vi "executePlayVSS.vi"(8 "error in (no error)":errorcluster, 11 "Game in":refnum<class "Game.lvclass">) -> (0 "error out":errorcluster, 3 "Game out":refnum<class "Game.lvclass">)   [LabVIEW 2020, in "Game.lvclass"]
uses:
  Game.lvclass
  Utilities_class/Utilities.lvclass
  HaltRole_class/HaltRole.lvclass
  AttackerAimGoalRoleVSS_class/AttackerAimGoalRoleVSS.lvclass
  Playbook_class/Playbook.lvclass
  BallChallengerAttackerRoleVSS_class/BallChallengerAttackerRoleVSS.lvclass
  KeeperRoleVSS_class/KeeperRoleVSS.lvclass
  NormalAttackerRoleVSS_class/NormalAttackerRoleVSS.lvclass
  DefenderAreaRoleVSS_class/DefenderAreaRoleVSS.lvclass
  TimeoutRole_class/TimeoutRole.lvclass
  PrepareFreeBallPlayVSS_class/PrepareFreeBallPlayVSS.lvclass
  PrepareGoalKickEnemyPlayVSS_class/PrepareGoalKickEnemyPlayVSS.lvclass
  Ally_class/Ally.lvclass
  TimeoutPlay_class/TimeoutPlay.lvclass
  DeadBallPlayVSS_class/DeadBallPlayVSS.lvclass
  NormalGamePlayVSS_class/NormalGamePlayVSS.lvclass
  PreparePenaltyAllyPlayVSS_class/PreparePenaltyAllyPlayVSS.lvclass
  HaltPlay_class/HaltPlay.lvclass
  BallChallengePlayVSS_class/BallChallengePlayVSS.lvclass
  PenaltyEnemyPlayVSS_class/PenaltyEnemyPlayVSS.lvclass
  KickPenaltyAllyPlayVSS_class/KickPenaltyAllyPlayVSS.lvclass
  Robot_class/Robot.lvclass
  PrepareGoalKickAllyPlayVSS_class/PrepareGoalKickAllyPlayVSS.lvclass
  PrepareKickoffAllyPlayVSS_class/PrepareKickoffAllyPlayVSS.lvclass
  PreparePenaltyEnemyPlayVSS_class/PreparePenaltyEnemyPlayVSS.lvclass
  PrepareKickoffEnemyPlay_class/PrepareKickoffEnemyPlay.lvclass
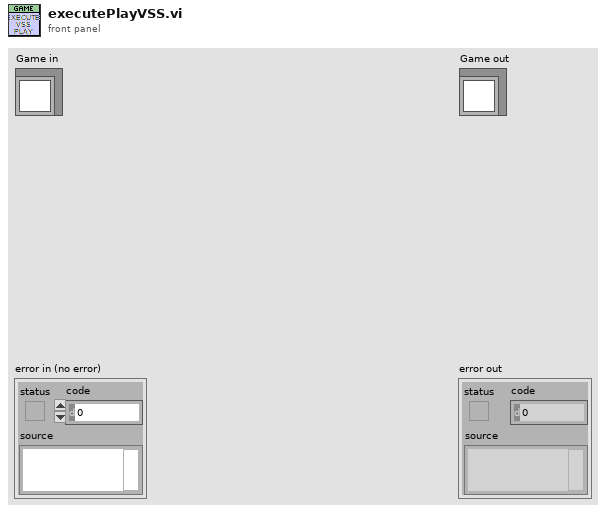
[diagram p1: front panel]
types:
  T1 = cluster{"id":i32, "x":dbl, "y":dbl, "orientation":dbl}[]
  T2 = enum16{"FreeBall", "PrepareFreeBall", "GoalKickEnemy", "GoalKickAlly", "KickoffAlly", "KickoffEnemy", "PrepareGoalKickEnemy", "PrepareGoalKickAlly", "Stop", "PrepareKickoffEnemy", "PrepareKickoffAlly", "PreparePenaltyEnemy", "Timeout", "DeadBall", "NormalGame", "KickPenaltyAlly", "PenaltyEnemy", "BallChallenge", "PreparePenaltyAlly", "Halt"}
  T3 = typedef "offensive_plays.ctl" = cluster{"Play":refnum<class "Play.lvclass">, "TestPlay":refnum<class "TestPlay.lvclass">, "EnemyPossessionAtEnemyFieldPlay":refnum<class "EnemyPossessionAtEnemyFieldPlay.lvclass">, "EnemyPossessionAtOurFieldPlay":refnum<class "EnemyPossessionAtOurFieldPlay.lvclass">, "NormalGamePlay":refnum<class "NormalGamePlay.lvclass">, "IndirectEnemyPlay":refnum<class "IndirectEnemyPlay.lvclass">, "PrepareKickoffAllyPlay":refnum<class "PrepareKickoffAllyPlay.lvclass">, "PrepareKickoffEnemyPlay":refnum<class "PrepareKickoffEnemyPlay.lvclass">, "KickPenaltyAllyPlay":refnum<class "KickPenaltyAllyPlay.lvclass">, "PreparePenaltyAllyPlay":refnum<class "PreparePenaltyAllyPlay.lvclass">, "DirectEnemyPlay":refnum<class "DirectEnemyPlay.lvclass">, "PreparePenaltyEnemyPlay":refnum<class "PreparePenaltyEnemyPlay.lvclass">, "BallOutOfFieldPlay":refnum<class "BallOutOfFieldPlay.lvclass">, "StopOffensivePlay":refnum<class "StopOffensivePlay.lvclass">, "PassPlay":refnum<class "PassPlay.lvclass">, "DirectKickPlay":refnum<class "DirectKickPlay.lvclass">, "HaltPlay":refnum<class "HaltPlay.lvclass">, "PreparePassPlay":refnum<class "PreparePassPlay.lvclass">, "PassToStrikerPlay":refnum<class "PassToStriker.lvclass">, "PassTo2ndStrikerPlay":refnum<class "PassTo2ndStriker.lvclass">, "SimplePassPlay":refnum<class "SimplePass.lvclass">, "PrepareRollToPassPlay":refnum<class "PrepareRollToPassPlay.lvclass">, "PrepareDoublePassPlay":refnum<class "PrepareDoublePassPlay.lvclass">, "TableWith2ndStrikerPlay":refnum<class "TableWith2ndStrikerPlay.lvclass">, "TableWithStrikerPlay":refnum<class "TableWithStrikerPlay.lvclass">}
  T4 = typedef "roles.ctl" = enum16{"BallChallengerAttackerVSS", "NormalAttackerVSS", "AttackerAimGoalVSS", "DefenderAreaVSS", "KeeperVSS", "Tabler", "TableFinalizer", "PrepareRollToPassRoller", "PrepareRollToPassReceiver", "SimplePassRoll", "SimplePassRollReceiver", "PenaltyDefense", "PreparePassReceiver 2", "PreparePassReceiver 1", "PassObserver", "Timeout", "Goto", "ZigZag", "None", "BallOutOfField", "DefenderArea", "Duelist", "AttackerStop", "FollowAttacker", "KeeperRole", "KickPenalty", "AttackerAimGoal", "AttackerBlock", "Marker", "Halt", "Shoot", "PassKicker", "PassReceiver", "TestRole", "PenaltyAttacker"}
  T5 = cluster{"HaltRole 1":refnum<class "HaltRole.lvclass">, "HaltRole 2":refnum<class "HaltRole.lvclass">, "HaltRole 3":refnum<class "HaltRole.lvclass">, "HaltRole 4":refnum<class "HaltRole.lvclass">, "HaltRole 5":refnum<class "HaltRole.lvclass">, "HaltRole 6":refnum<class "HaltRole.lvclass">}
  T6 = cluster{"PreparePenaltyAllyPlayVSS":refnum<class "PreparePenaltyAllyPlayVSS.lvclass">, "HaltPlay":refnum<class "HaltPlay.lvclass">, "DeadBallPlayVSS":refnum<class "DeadBallPlayVSS.lvclass">, "NormalGamePlayVSS":refnum<class "NormalGamePlayVSS.lvclass">, "BallChallengePlayVSS":refnum<class "BallChallengePlayVSS.lvclass">, "PenaltyEnemyPlayVSS":refnum<class "PenaltyEnemyPlayVSS.lvclass">, "TimeoutPlay":refnum<class "TimeoutPlay.lvclass">, "KickPenaltyAllyPlayVSS":refnum<class "KickPenaltyAllyPlayVSS.lvclass">, "PreparePenaltyEnemyPlayVSS":refnum<class "PreparePenaltyEnemyPlayVSS.lvclass">, "PrepareKickoffAllyPlayVSS":refnum<class "PrepareKickoffAllyPlayVSS.lvclass">, "PrepareKickoffEnemyPlayVSS":refnum<class "PrepareKickoffEnemyPlayVSS.lvclass">, "PrepareGoalKickAllyPlayVSS":refnum<class "PrepareGoalKickAllyPlayVSS.lvclass">, "PrepareGoalKickEnemyPlayVSS":refnum<class "PrepareGoalKickEnemyPlayVSS.lvclass">, "PrepareFreeBallPlayVSS":refnum<class "PrepareFreeBallPlayVSS.lvclass">, "FreeBallPlayVSS":refnum<class "FreeBallPlayVSS.lvclass">, "GoalKickAllyPlayVSS":refnum<class "GoalKickAllyPlayVSS.lvclass">, "GoalKickEnemyPlayVSS":refnum<class "GoalKickEnemyPlayVSS.lvclass">, "KickoffAllyPlayVSS":refnum<class "KickoffAllyPlayVSS.lvclass">, "KickoffEnemyPlayVSS":refnum<class "KickoffEnemyPlayVSS.lvclass">, "StopPlayVSS":refnum<class "StopPlayVSS.lvclass">}
  T7 = cluster{"HaltRole 1":refnum<class "HaltRole.lvclass">, "HaltRole 2":refnum<class "HaltRole.lvclass">, "AttackerAimGoalRoleVSS":refnum<class "AttackerAimGoalRoleVSS.lvclass">}
  T8 = cluster{"HaltRole 1":refnum<class "HaltRole.lvclass">, "HaltRole 2":refnum<class "HaltRole.lvclass">, "BallChallengerAttackerRoleVSS":refnum<class "BallChallengerAttackerRoleVSS.lvclass">}
  T9 = cluster{"KeeperRoleVSS":refnum<class "KeeperRoleVSS.lvclass">, "HaltRole 1":refnum<class "HaltRole.lvclass">, "HaltRole 2":refnum<class "HaltRole.lvclass">}
  T10 = cluster{"NormalAttackerRoleVSS":refnum<class "NormalAttackerRoleVSS.lvclass">, "HaltRole 1":refnum<class "HaltRole.lvclass">, "HaltRole 2":refnum<class "HaltRole.lvclass">}
  T11 = cluster{"NormalAttackerRoleVSS":refnum<class "NormalAttackerRoleVSS.lvclass">, "KeeperRoleVSS":refnum<class "KeeperRoleVSS.lvclass">, "DefenderAreaRoleVSS":refnum<class "DefenderAreaRoleVSS.lvclass">}
  T12 = cluster{"TimeoutRole 1":refnum<class "TimeoutRole.lvclass">, "TimeoutRole 2":refnum<class "TimeoutRole.lvclass">, "TimeoutRole 3":refnum<class "TimeoutRole.lvclass">, "TimeoutRole 4":refnum<class "TimeoutRole.lvclass">, "TimeoutRole 5":refnum<class "TimeoutRole.lvclass">, "TimeoutRole 6":refnum<class "TimeoutRole.lvclass">}
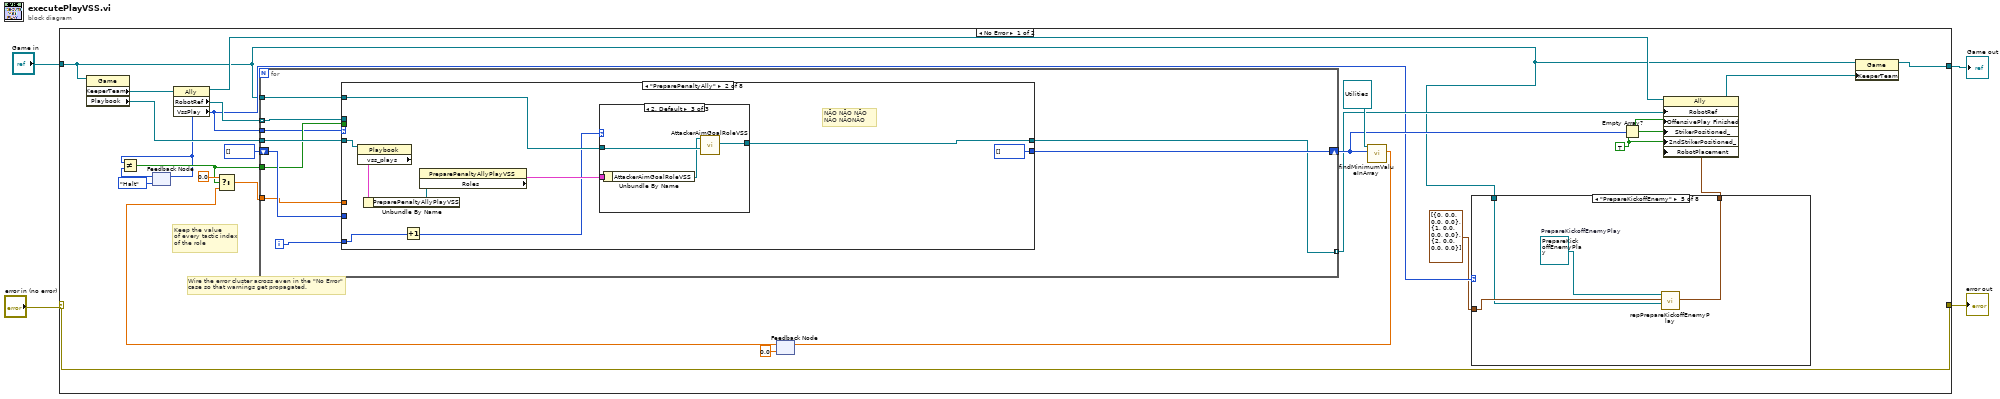
[diagram p0: block diagram]
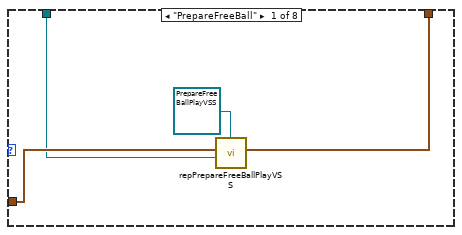
[diagram p2: hidden frame]
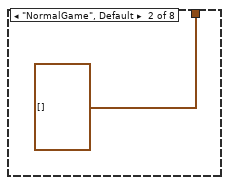
[diagram p3: hidden frame]
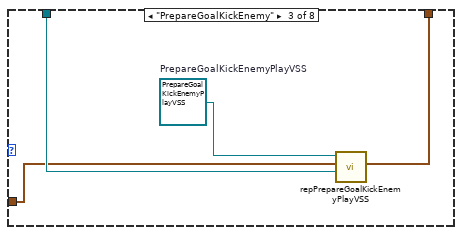
[diagram p4: hidden frame]
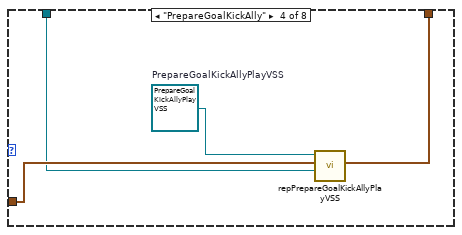
[diagram p5: hidden frame]
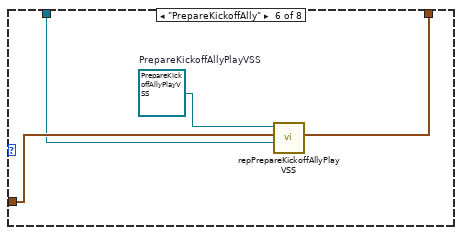
[diagram p6: hidden frame]
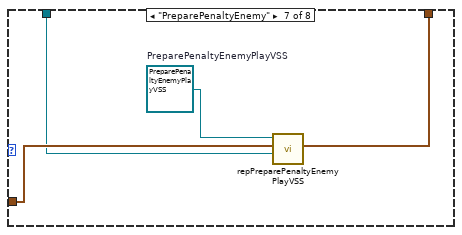
[diagram p7: hidden frame]
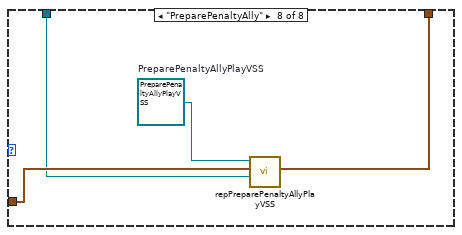
[diagram p8: hidden frame]
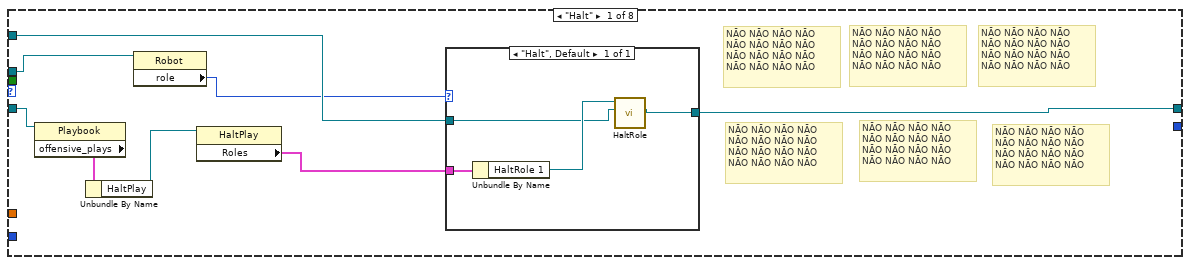
[diagram p9: hidden frame]
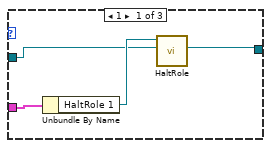
[diagram p10: hidden frame]
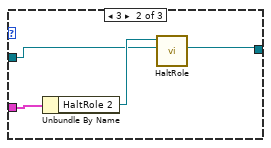
[diagram p11: hidden frame]
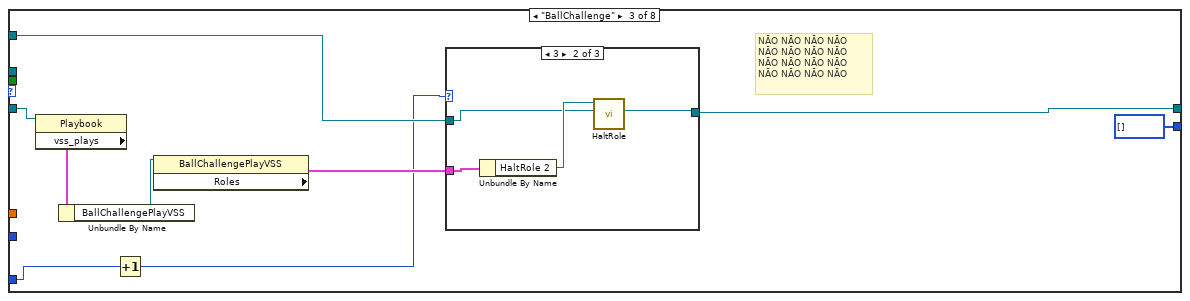
[diagram p12: hidden frame]
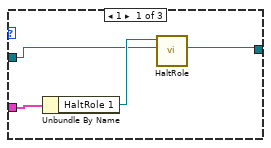
[diagram p13: hidden frame]
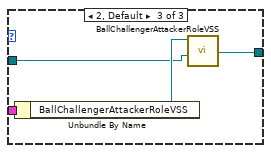
[diagram p14: hidden frame]
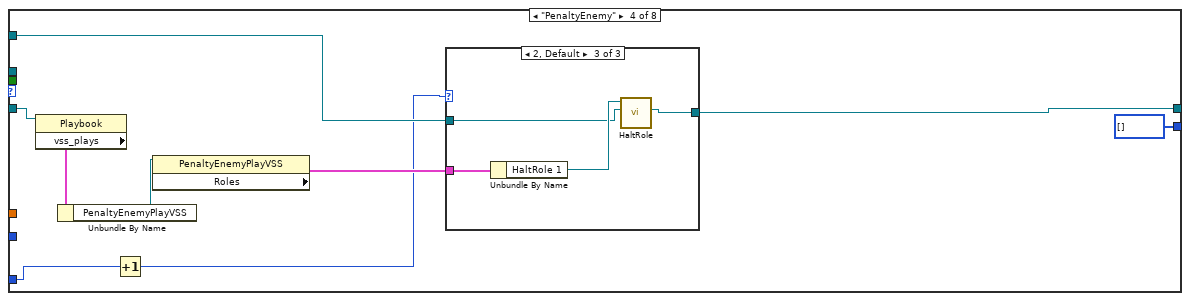
[diagram p15: hidden frame]
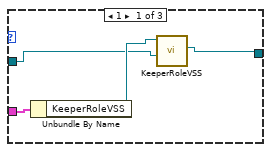
[diagram p16: hidden frame]
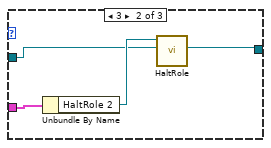
[diagram p17: hidden frame]
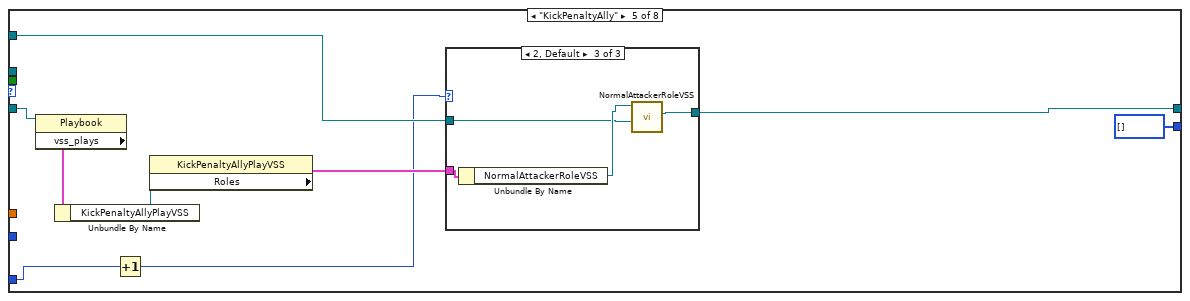
[diagram p18: hidden frame]
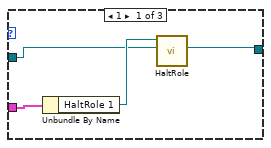
[diagram p19: hidden frame]
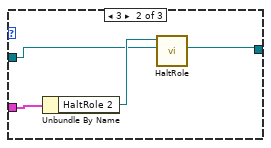
[diagram p20: hidden frame]
diagram:
  n1 = case shown="No Error" "error in (no error)" {
    selector: "error in (no error)" -> [w29 w236]
    tunnel: [w29 w236] -> w3
    tunnel: [w7 w235] -> w4
    tunnel: "Game in" -> [w8 w235]
    frame No Error {
      w14 = TRUE
      # "Keep the value\nof every tactic index\nof the role"
      # "Wire the error cluster across even in the \"No Error\"\ncase so that warnings get propagated."
      n2 = property class="Game"(reference=w8) -> ("KeeperTeam"=w28:refnum<class "Ally.lvclass">, "Playbook"=w26:refnum<class "Playbook.lvclass">)  [unwired: 1 in, 2 out]
      n3 = feedback #1(T2."Halt" ("VssPlay")) -> (w21:T2)
      n4 = property class="Ally"(reference=w28) -> (reference out=w12:refnum<class "Ally.lvclass">, "RobotRef"=w27:refnum<class "Robot.lvclass">[], "VssPlay"=w9:T2)  [unwired: 1 in, 1 out]
      n5 = Not Equal?(x=w9, y=w21) -> (x != y?=w18:bool)
      n6 = feedback-in #1(w9) -> ()
      n7 = feedback #2(0.0 ("minimum")) -> (w20:dbl)
      n8 = Select(t=0.0, s=w18, f=w20) -> (s? t:f=w13:dbl)
      n9 = for {
        tunnel: w27 -> [w63] mode=indexing
        tunnel: w26 -> [w68]
        tunnel: w8 -> [w67]
        shift-right: [w66] -> w16
        shift-left: i32[] [] -> [w65]
        tunnel: w18 -> [w64]
        tunnel: w13 -> [w62]
        tunnel: [w60] -> w11 mode=indexing
        tunnel: w9 -> [w59]
        i -> [w61]
        n10 = case shown="\"PreparePenaltyAlly\"" w59 {
          tunnel: w68 -> [w76 w89 w110 w131 w152 w174 w197 w219]
          tunnel: w67 -> [w72 w85 w106 w127 w148 w170 w193 w215]
          tunnel: [w71 w84 w105 w126 w147 w169 w192 w214] -> w60
          tunnel: w62 -> [_ _ _ _ _ _ _ _]
          tunnel: [_ i32[] [] i32[] [] i32[] [] i32[] [] i32[] [] i32[] [] i32[] []] -> w66
          tunnel: w65 -> [_ _ _ _ _ _ _ _]
          tunnel: w64 -> [_ _ _ _ _ w165 _ _]
          tunnel: w63 -> [w70 _ _ _ _ _ _ w210]
          tunnel: w61 -> [_ w82 w103 w124 w145 w167 w190 w212]
          frame "Halt" {
            # "NÃO NÃO NÃO NÃO\nNÃO NÃO NÃO NÃO\nNÃO NÃO NÃO NÃO\nNÃO NÃO NÃO NÃO"
            # "NÃO NÃO NÃO NÃO\nNÃO NÃO NÃO NÃO\nNÃO NÃO NÃO NÃO\nNÃO NÃO NÃO NÃO"
            # "NÃO NÃO NÃO NÃO\nNÃO NÃO NÃO NÃO\nNÃO NÃO NÃO NÃO\nNÃO NÃO NÃO NÃO"
            # "NÃO NÃO NÃO NÃO\nNÃO NÃO NÃO NÃO\nNÃO NÃO NÃO NÃO\nNÃO NÃO NÃO NÃO"
            # "NÃO NÃO NÃO NÃO\nNÃO NÃO NÃO NÃO\nNÃO NÃO NÃO NÃO\nNÃO NÃO NÃO NÃO"
            # "NÃO NÃO NÃO NÃO\nNÃO NÃO NÃO NÃO\nNÃO NÃO NÃO NÃO\nNÃO NÃO NÃO NÃO"
            n11 = property class="Playbook"(reference=w76) -> ("offensive_plays"=w75:T3)  [unwired: 1 in, 2 out]
            n12 = Unbundle By Name(w75) -> ("HaltPlay"=w74:refnum<class "HaltPlay.lvclass">)
            n13 = property class="Robot"(reference=w70) -> ("role"=w69:T4)  [unwired: 1 in, 2 out]
            n14 = property class="HaltPlay"(reference=w74) -> ("Roles"=w73:T5)  [unwired: 1 in, 2 out]
            n15 = case shown="\"Halt\", Default" w69 {
              tunnel: w73 -> [w80]
              tunnel: w72 -> [w78]
              tunnel: [w77] -> w71
              frame "Halt", Default {
                n16 = Unbundle By Name(w80) -> ("HaltRole 1"=w79:refnum<class "HaltRole.lvclass">)
                n17 = call "HaltRole.vi"("Game in"=w78, "HaltRole in"=w79) -> ("Robot out"=w77:refnum<class "Robot.lvclass">)  [unwired: 6 in, 3 out]
              }
            }
          }
          frame "PreparePenaltyAlly" {
            # "NÃO NÃO NÃO \nNÃO NÃONÃO"
            n18 = property class="Playbook"(reference=w89) -> ("vss_plays"=w88:T6)  [unwired: 1 in, 2 out]
            n19 = Unbundle By Name(w88) -> ("PreparePenaltyAllyPlayVSS"=w87:refnum<class "PreparePenaltyAllyPlayVSS.lvclass">)
            n20 = Increment(x=w82) -> (x+1=w81:i32)
            n21 = property class="PreparePenaltyAllyPlayVSS"(reference=w87) -> ("Roles"=w86:T7)  [unwired: 1 in, 2 out]
            n22 = case shown="2, Default" w81 {
              tunnel: w86 -> [w93 w97 w101]
              tunnel: w85 -> [w91 w95 w99]
              tunnel: [w90 w94 w100] -> w84
              frame 1 {
                n23 = Unbundle By Name(w93) -> ("HaltRole 1"=w92:refnum<class "HaltRole.lvclass">)
                n24 = call "HaltRole.vi"("Game in"=w91, "HaltRole in"=w92) -> ("Robot out"=w90:refnum<class "Robot.lvclass">)  [unwired: 6 in, 3 out]
              }
              frame 3 {
                n25 = Unbundle By Name(w97) -> ("HaltRole 2"=w96:refnum<class "HaltRole.lvclass">)
                n26 = call "HaltRole.vi"("Game in"=w95, "HaltRole in"=w96) -> ("Robot out"=w94:refnum<class "Robot.lvclass">)  [unwired: 6 in, 3 out]
              }
              frame 2, Default {
                n27 = Unbundle By Name(w101) -> ("AttackerAimGoalRoleVSS"=w98:refnum<class "AttackerAimGoalRoleVSS.lvclass">)
                n28 = call "AttackerAimGoalRoleVSS.vi"("Game in"=w99, "AttackerAimGoalRoleVSS in"=w98) -> ("Robot out"=w100:refnum<class "Robot.lvclass">)  [unwired: 6 in, 3 out]
              }
            }
          }
          frame "BallChallenge" {
            # "NÃO NÃO NÃO NÃO\nNÃO NÃO NÃO NÃO\nNÃO NÃO NÃO NÃO\nNÃO NÃO NÃO NÃO"
            n29 = property class="Playbook"(reference=w110) -> ("vss_plays"=w109:T6)  [unwired: 1 in, 2 out]
            n30 = Unbundle By Name(w109) -> ("BallChallengePlayVSS"=w108:refnum<class "BallChallengePlayVSS.lvclass">)
            n31 = Increment(x=w103) -> (x+1=w102:i32)
            n32 = property class="BallChallengePlayVSS"(reference=w108) -> ("Roles"=w107:T8)  [unwired: 1 in, 2 out]
            n33 = case shown="3" w102 {
              tunnel: w107 -> [w114 w118 w122]
              tunnel: w106 -> [w112 w116 w119]
              tunnel: [w111 w115 w121] -> w105
              frame 1 {
                n34 = Unbundle By Name(w114) -> ("HaltRole 1"=w113:refnum<class "HaltRole.lvclass">)
                n35 = call "HaltRole.vi"("Game in"=w112, "HaltRole in"=w113) -> ("Robot out"=w111:refnum<class "Robot.lvclass">)  [unwired: 6 in, 3 out]
              }
              frame 3 {
                n36 = Unbundle By Name(w118) -> ("HaltRole 2"=w117:refnum<class "HaltRole.lvclass">)
                n37 = call "HaltRole.vi"("Game in"=w116, "HaltRole in"=w117) -> ("Robot out"=w115:refnum<class "Robot.lvclass">)  [unwired: 6 in, 3 out]
              }
              frame 2, Default {
                n38 = Unbundle By Name(w122) -> ("BallChallengerAttackerRoleVSS"=w120:refnum<class "BallChallengerAttackerRoleVSS.lvclass">)
                n39 = call "BallChallengerAttackerRoleVSS.vi"("Game in"=w119, "BallChallengerAttackerRoleVSS in"=w120) -> ("Robot out"=w121:refnum<class "Robot.lvclass">)  [unwired: 6 in, 3 out]
              }
            }
          }
          frame "PenaltyEnemy" {
            n40 = property class="Playbook"(reference=w131) -> ("vss_plays"=w130:T6)  [unwired: 1 in, 2 out]
            n41 = Unbundle By Name(w130) -> ("PenaltyEnemyPlayVSS"=w129:refnum<class "PenaltyEnemyPlayVSS.lvclass">)
            n42 = Increment(x=w124) -> (x+1=w123:i32)
            n43 = property class="PenaltyEnemyPlayVSS"(reference=w129) -> ("Roles"=w128:T9)  [unwired: 1 in, 2 out]
            n44 = case shown="2, Default" w123 {
              tunnel: w128 -> [w135 w139 w143]
              tunnel: w127 -> [w132 w137 w141]
              tunnel: [w134 w136 w140] -> w126
              frame 1 {
                n45 = Unbundle By Name(w135) -> ("KeeperRoleVSS"=w133:refnum<class "KeeperRoleVSS.lvclass">)
                n46 = call "KeeperRoleVSS.vi"("Game in"=w132, "KeeperRoleVSS in"=w133) -> ("Robot out"=w134:refnum<class "Robot.lvclass">)  [unwired: 6 in, 3 out]
              }
              frame 3 {
                n47 = Unbundle By Name(w139) -> ("HaltRole 2"=w138:refnum<class "HaltRole.lvclass">)
                n48 = call "HaltRole.vi"("Game in"=w137, "HaltRole in"=w138) -> ("Robot out"=w136:refnum<class "Robot.lvclass">)  [unwired: 6 in, 3 out]
              }
              frame 2, Default {
                n49 = Unbundle By Name(w143) -> ("HaltRole 1"=w142:refnum<class "HaltRole.lvclass">)
                n50 = call "HaltRole.vi"("Game in"=w141, "HaltRole in"=w142) -> ("Robot out"=w140:refnum<class "Robot.lvclass">)  [unwired: 6 in, 3 out]
              }
            }
          }
          frame "KickPenaltyAlly" {
            n51 = property class="Playbook"(reference=w152) -> ("vss_plays"=w151:T6)  [unwired: 1 in, 2 out]
            n52 = Unbundle By Name(w151) -> ("KickPenaltyAllyPlayVSS"=w150:refnum<class "KickPenaltyAllyPlayVSS.lvclass">)
            n53 = Increment(x=w145) -> (x+1=w144:i32)
            n54 = property class="KickPenaltyAllyPlayVSS"(reference=w150) -> ("Roles"=w149:T10)  [unwired: 1 in, 2 out]
            n55 = case shown="2, Default" w144 {
              tunnel: w149 -> [w156 w160 w164]
              tunnel: w148 -> [w154 w158 w162]
              tunnel: [w153 w157 w161] -> w147
              frame 1 {
                n56 = Unbundle By Name(w156) -> ("HaltRole 1"=w155:refnum<class "HaltRole.lvclass">)
                n57 = call "HaltRole.vi"("Game in"=w154, "HaltRole in"=w155) -> ("Robot out"=w153:refnum<class "Robot.lvclass">)  [unwired: 6 in, 3 out]
              }
              frame 3 {
                n58 = Unbundle By Name(w160) -> ("HaltRole 2"=w159:refnum<class "HaltRole.lvclass">)
                n59 = call "HaltRole.vi"("Game in"=w158, "HaltRole in"=w159) -> ("Robot out"=w157:refnum<class "Robot.lvclass">)  [unwired: 6 in, 3 out]
              }
              frame 2, Default {
                n60 = Unbundle By Name(w164) -> ("NormalAttackerRoleVSS"=w163:refnum<class "NormalAttackerRoleVSS.lvclass">)
                n61 = call "NormalAttackerRoleVSS.vi"("Game in"=w162, "NormalAttackerRoleVSS in"=w163) -> ("Robot out"=w161:refnum<class "Robot.lvclass">)  [unwired: 6 in, 3 out]
              }
            }
          }
          frame "NormalGame", Default {
            n62 = property class="Playbook"(reference=w174) -> ("vss_plays"=w173:T6)  [unwired: 1 in, 2 out]
            n63 = Unbundle By Name(w173) -> ("NormalGamePlayVSS"=w172:refnum<class "NormalGamePlayVSS.lvclass">)
            n64 = Increment(x=w167) -> (x+1=w166:i32)
            n65 = property class="NormalGamePlayVSS"(reference=w172) -> ("Roles"=w171:T11)  [unwired: 1 in, 2 out]
            n66 = case shown="3" w166 {
              tunnel: w171 -> [w178 w183 w188]
              tunnel: w170 -> [w176 w181 w186]
              tunnel: [w175 w180 w185] -> w169
              tunnel: w165 -> [_ w179 w184]
              frame 1, Default {
                n67 = Unbundle By Name(w178) -> ("KeeperRoleVSS"=w177:refnum<class "KeeperRoleVSS.lvclass">)
                n68 = call "KeeperRoleVSS.vi"("Game in"=w176, "KeeperRoleVSS in"=w177) -> ("Robot out"=w175:refnum<class "Robot.lvclass">)  [unwired: 6 in, 3 out]
              }
              frame 3 {
                n69 = Unbundle By Name(w183) -> ("DefenderAreaRoleVSS"=w182:refnum<class "DefenderAreaRoleVSS.lvclass">)
                n70 = call "DefenderAreaRoleVSS.vi"("First call?"=w179, "Game in"=w181, "DefenderAreaRoleVSS in"=w182) -> ("Robot out"=w180:refnum<class "Robot.lvclass">)  [unwired: 5 in, 3 out]
              }
              frame 2 {
                n71 = Unbundle By Name(w188) -> ("NormalAttackerRoleVSS"=w187:refnum<class "NormalAttackerRoleVSS.lvclass">)
                n72 = call "NormalAttackerRoleVSS.vi"("First call?"=w184, "Game in"=w186, "NormalAttackerRoleVSS in"=w187) -> ("Robot out"=w185:refnum<class "Robot.lvclass">)  [unwired: 5 in, 3 out]
              }
            }
          }
          frame "DeadBall" {
            # "NÃO NÃO NÃO NÃO\nNÃO NÃO NÃO NÃO\nNÃO NÃO NÃO NÃO\nNÃO NÃO NÃO NÃO"
            n73 = property class="Playbook"(reference=w197) -> ("vss_plays"=w196:T6)  [unwired: 1 in, 2 out]
            n74 = Unbundle By Name(w196) -> ("DeadBallPlayVSS"=w195:refnum<class "DeadBallPlayVSS.lvclass">)
            n75 = Increment(x=w190) -> (x+1=w189:i32)
            n76 = property class="DeadBallPlayVSS"(reference=w195) -> ("Roles"=w194:T11)  [unwired: 1 in, 2 out]
            n77 = case shown="3" w189 {
              tunnel: w194 -> [w201 w205 w209]
              tunnel: w193 -> [w199 w203 w207]
              tunnel: [w198 w202 w206] -> w192
              frame 1 {
                n78 = Unbundle By Name(w201) -> ("KeeperRoleVSS"=w200:refnum<class "KeeperRoleVSS.lvclass">)
                n79 = call "KeeperRoleVSS.vi"("Game in"=w199, "KeeperRoleVSS in"=w200) -> ("Robot out"=w198:refnum<class "Robot.lvclass">)  [unwired: 6 in, 3 out]
              }
              frame 3 {
                n80 = Unbundle By Name(w205) -> ("DefenderAreaRoleVSS"=w204:refnum<class "DefenderAreaRoleVSS.lvclass">)
                n81 = call "DefenderAreaRoleVSS.vi"("Game in"=w203, "DefenderAreaRoleVSS in"=w204) -> ("Robot out"=w202:refnum<class "Robot.lvclass">)  [unwired: 6 in, 3 out]
              }
              frame 2, Default {
                n82 = Unbundle By Name(w209) -> ("NormalAttackerRoleVSS"=w208:refnum<class "NormalAttackerRoleVSS.lvclass">)
                n83 = call "NormalAttackerRoleVSS.vi"("Game in"=w207, "NormalAttackerRoleVSS in"=w208) -> ("Robot out"=w206:refnum<class "Robot.lvclass">)  [unwired: 6 in, 3 out]
              }
            }
          }
          frame "Timeout" {
            # "NÃO NÃO NÃO NÃO\nNÃO NÃO NÃO NÃO\nNÃO NÃO NÃO NÃO\nNÃO NÃO NÃO NÃO"
            n84 = property class="Playbook"(reference=w219) -> ("vss_plays"=w218:T6)  [unwired: 1 in, 2 out]
            n85 = Unbundle By Name(w218) -> ("TimeoutPlay"=w217:refnum<class "TimeoutPlay.lvclass">)
            n86 = Increment(x=w212) -> (x+1=w211:i32)
            n87 = property class="TimeoutPlay"(reference=w217) -> ("Roles"=w216:T12)  [unwired: 1 in, 2 out]
            n88 = case shown="3" w211 {
              tunnel: w216 -> [w224 w229 w234]
              tunnel: w215 -> [w222 w227 w232]
              tunnel: [w221 w226 w231] -> w214
              tunnel: w210 -> [w220 w225 w230]
              frame 1, Default {
                n89 = Unbundle By Name(w224) -> ("TimeoutRole 1"=w223:refnum<class "TimeoutRole.lvclass">)
                n90 = call-dynamic "TimeoutRole.vi"("Game in"=w222, "Robot in"=w220, "TimeoutRole in"=w223) -> ("Robot out"=w221:refnum<class "Robot.lvclass">)  [unwired: 5 in, 3 out]
              }
              frame 2 {
                n91 = Unbundle By Name(w229) -> ("TimeoutRole 2"=w228:refnum<class "TimeoutRole.lvclass">)
                n92 = call-dynamic "TimeoutRole.vi"("Game in"=w227, "Robot in"=w225, "TimeoutRole in"=w228) -> ("Robot out"=w226:refnum<class "Robot.lvclass">)  [unwired: 5 in, 3 out]
              }
              frame 3 {
                n93 = Unbundle By Name(w234) -> ("TimeoutRole 3"=w233:refnum<class "TimeoutRole.lvclass">)
                n94 = call-dynamic "TimeoutRole.vi"("Game in"=w232, "Robot in"=w230, "TimeoutRole in"=w233) -> ("Robot out"=w231:refnum<class "Robot.lvclass">)  [unwired: 5 in, 3 out]
              }
            }
          }
        }
      }
      n95 = call-dynamic "findMinimumValueInArray.vi"("array"=w16, "Utilities in"=refnum<class "Utilities.lvclass"> refnum) -> ("minimum"=w23:dbl)  [unwired: 7 in, 2 out]
      n96 = feedback-in #2(w23) -> ()
      n97 = case shown="\"PrepareKickoffEnemy\"" w9 {
        tunnel: w8 -> [w30 _ w36 w41 w43 w48 w53 w56]
        tunnel: [w31 T1 [] ("RobotPlacement") w37 w39 w45 w47 w51 w55] -> w5
        tunnel: T1 [{"id"=0, "x"=0.0, "y"=0.0, "orientation"=0.0}, {"id"=1, "x"=0.0, "y"=0.0, "orientation"=0.0}, {"id"=2, "x"=0.0, "y"=0.0, "orientation"=0.0}] ("RobotPlacement") -> [w32 _ w35 w42 w44 w49 w54 w57]
        frame "PrepareFreeBall" {
          n98 = call "repPrepareFreeBallPlayVSS.vi"("Game in 2"=w30, "RobotPlacement"=w32, "PrepareFreeBallPlayVSS in"=refnum<class "PrepareFreeBallPlayVSS.lvclass"> refnum) -> ("RobotPlacement 2"=w31:T1)  [unwired: 6 in, 2 out]
        }
        frame "NormalGame", Default {
        }
        frame "PrepareGoalKickEnemy" {
          w38 = refnum<class "PrepareGoalKickEnemyPlayVSS.lvclass"> refnum  # PrepareGoalKickEnemyPlayVSS
          n99 = call "repPrepareGoalKickEnemyPlayVSS.vi"("PrepareGoalKickEnemyPlayVSS in"=w38, "RobotPlacement"=w35, "Game in 2"=w36) -> ("RobotPlacement 2"=w37:T1)  [unwired: 5 in, 2 out]
        }
        frame "PrepareGoalKickAlly" {
          w40 = refnum<class "PrepareGoalKickAllyPlayVSS.lvclass"> refnum  # PrepareGoalKickAllyPlayVSS
          n100 = call "repPrepareGoalKickAllyPlayVSS.vi"("Game in 2"=w41, "RobotPlacement"=w42, "PrepareGoalKickAllyPlayVSS in"=w40) -> ("RobotPlacement 2"=w39:T1)  [unwired: 6 in, 2 out]
        }
        frame "PrepareKickoffEnemy" {
          w46 = refnum<class "PrepareKickoffEnemyPlay.lvclass"> refnum  # PrepareKickoffEnemyPlay
          n101 = call "repPrepareKickoffEnemyPlay.vi"("Game in 2"=w43, "RobotPlacement"=w44, "PrepareKickoffEnemyPlay in"=w46) -> ("RobotPlacement 2"=w45:T1)  [unwired: 6 in, 2 out]
        }
        frame "PrepareKickoffAlly" {
          w50 = refnum<class "PrepareKickoffAllyPlayVSS.lvclass"> refnum  # PrepareKickoffAllyPlayVSS
          n102 = call "repPrepareKickoffAllyPlayVSS.vi"("Game in 2"=w48, "RobotPlacement"=w49, "PrepareKickoffAllyPlayVSS in"=w50) -> ("RobotPlacement 2"=w47:T1)  [unwired: 6 in, 2 out]
        }
        frame "PreparePenaltyEnemy" {
          w52 = refnum<class "PreparePenaltyEnemyPlayVSS.lvclass"> refnum  # PreparePenaltyEnemyPlayVSS
          n103 = call "repPreparePenaltyEnemyPlayVSS.vi"("Game in 2"=w53, "RobotPlacement"=w54, "PreparePenaltyEnemyPlayVSS in"=w52) -> ("RobotPlacement 2"=w51:T1)  [unwired: 6 in, 2 out]
        }
        frame "PreparePenaltyAlly" {
          w58 = refnum<class "PreparePenaltyAllyPlayVSS.lvclass"> refnum  # PreparePenaltyAllyPlayVSS
          n104 = call "repPreparePenaltyAllyPlayVSS.vi"("Game in 2"=w56, "RobotPlacement"=w57, "PreparePenaltyAllyPlayVSS in"=w58) -> ("RobotPlacement 2"=w55:T1)  [unwired: 6 in, 2 out]
        }
      }
      n105 = Empty Array?(array=w16) -> (empty?=w17:bool)
      n106 = property class="Ally"(reference=w12, "RobotRef"=w11, "OffensivePlay Finished"=w17, "StrikerPositioned_"=w14, "2ndStrikerPositioned_"=w14, "RobotPlacement"=w5) -> (reference out=w25:refnum<class "Ally.lvclass">)  [unwired: 1 in, 1 out]
      n107 = property class="Game"(reference=w8, "KeeperTeam"=w25) -> (reference out=w7:refnum<class "Game.lvclass">)  [unwired: 1 in, 1 out]
    }
    frame Error {
    }
  }
  "error out" <- w3
  "Game out" <- w4
